vi "Read Report File Name.vi"(8 "error in (no error)":errorcluster, 11 "XML Report In":refnum<class "XML Report.lvclass">) -> (0 "error out":errorcluster, 1 "Report File Name without extension":string, 2 "Report Name":string, 3 "XML Report Out":refnum<class "XML Report.lvclass">)   [LabVIEW 2020, in "XML Report.lvclass"]
uses:
  XML Report.lvclass
  Test Report/Test Report.lvclass
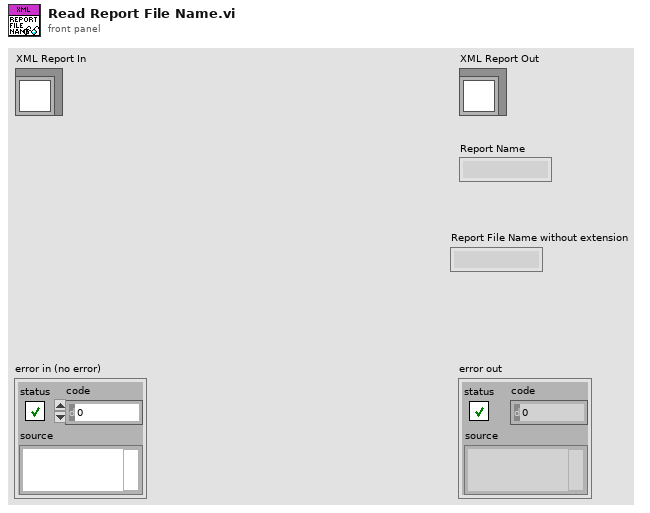
[diagram p1: front panel]
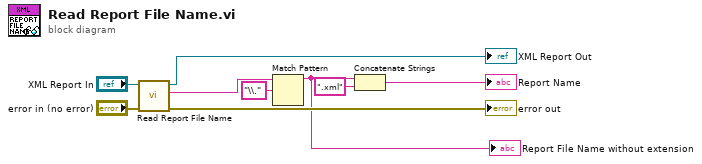
[diagram p0: block diagram]
diagram:
  n1 = call-parent "Read Report File Name.vi"("error in (no error)"="error in (no error)", "Report In"="XML Report In") -> ("error out"=→"error out":errorcluster, "Report File Name"=w2:string, "Report Out"=→"XML Report Out":refnum<class "XML Report.lvclass">)  [unwired: 6 in, 1 out]
  n2 = Match Pattern(string=w2, regular expression="\\.") -> (before substring=w1:string)  [unwired: 1 in, 3 out]
  "Report File Name without extension" <- w1
  n3 = Concatenate Strings(w1, ".xml" ("string")) -> (→"Report Name":string)
